vi "Python과 TCP 연결하여 드론 날리기.vi"() -> ()   [LabVIEW 2025]
panel:
  in  "read byte":u32
  in  "port":u32
  in  "localhost":string
  in  "뒤로 플립":bool
  in  "오른쪽 플립":bool
  in  "왼쪽 플립":bool
  in  "우측 회전":bool
  in  "좌측 회전":bool
  in  "하강":bool
  in  "상승":bool
  in  "리턴 홈":bool
  in  "후진":bool
  in  "우측 이동":bool
  in  "좌측 이동":bool
  in  "착륙":bool
  in  "앞으로 플립":bool
  in  "전진":bool
  out "결과":string
  in  "이륙":bool
  in  "종료":bool
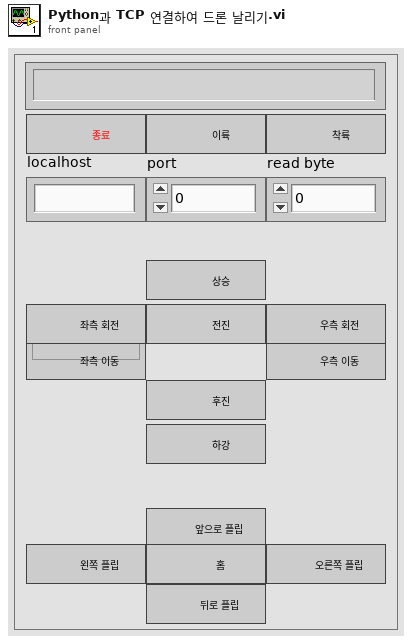
[diagram p1: front panel]
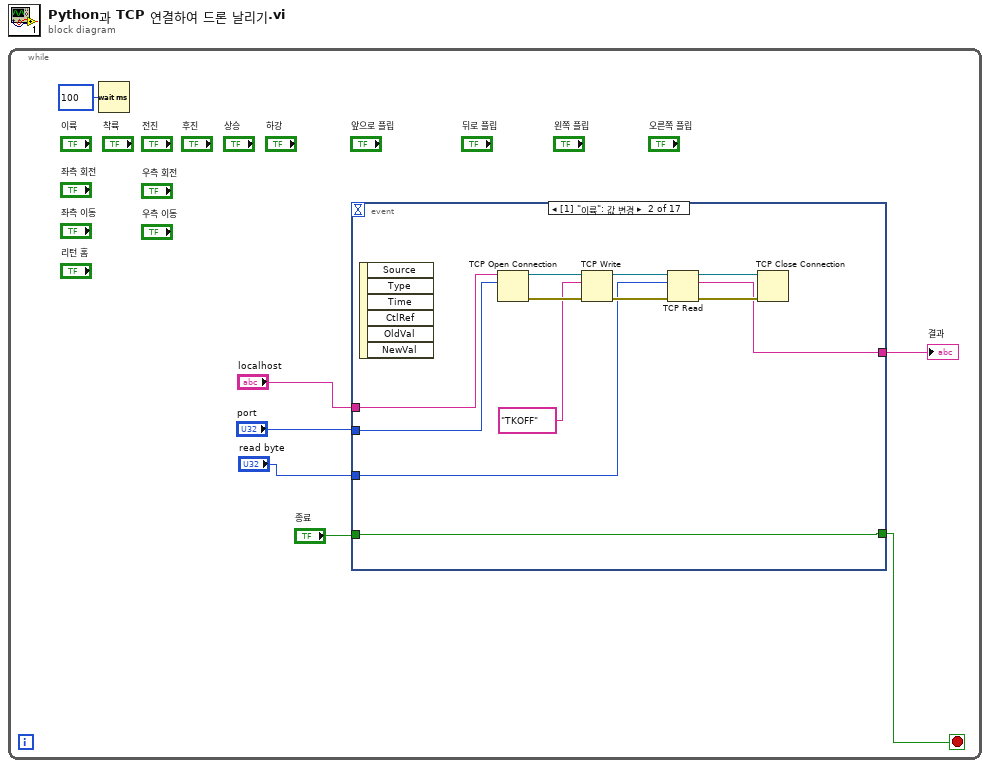
[diagram p0: block diagram]
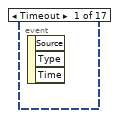
[diagram p2: hidden frame]
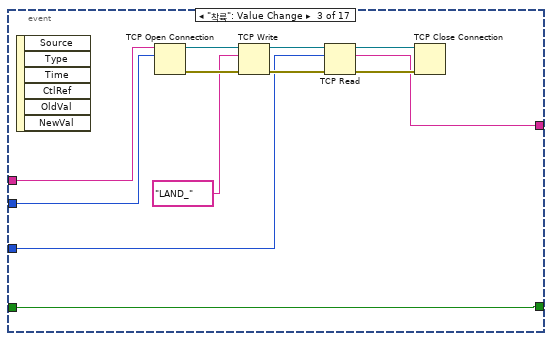
[diagram p3: hidden frame]
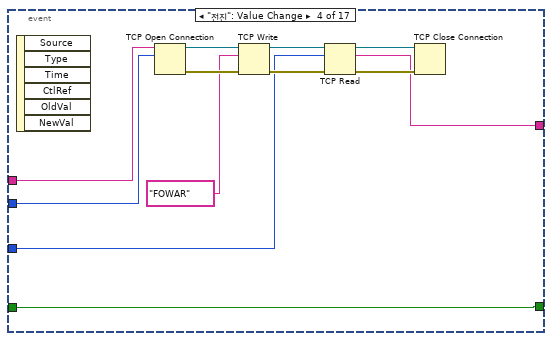
[diagram p4: hidden frame]
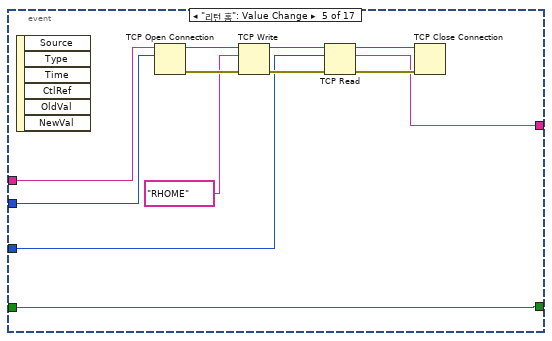
[diagram p5: hidden frame]
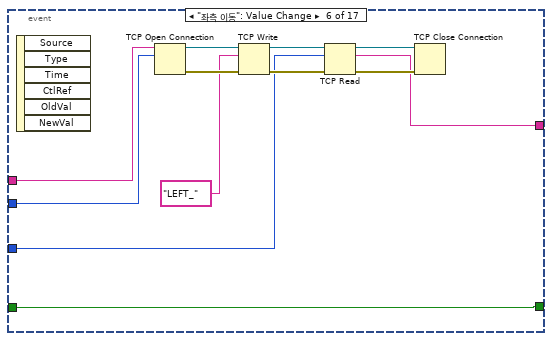
[diagram p6: hidden frame]
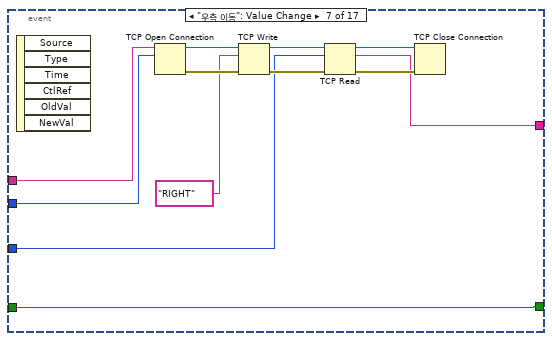
[diagram p7: hidden frame]
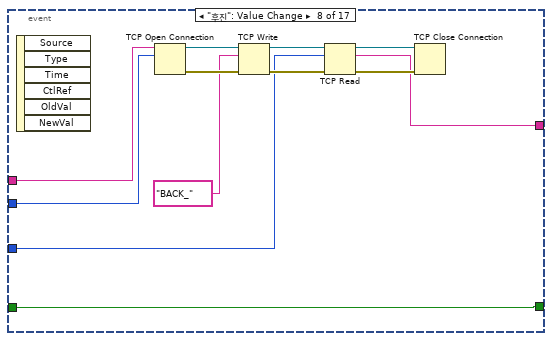
[diagram p8: hidden frame]
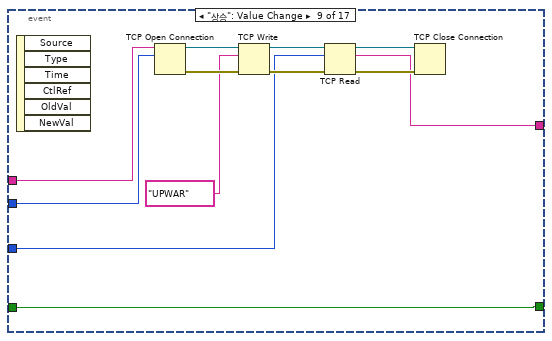
[diagram p9: hidden frame]
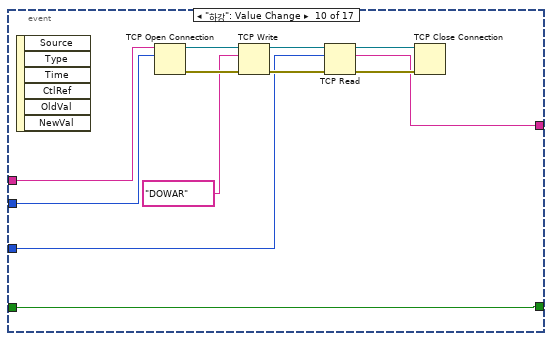
[diagram p10: hidden frame]
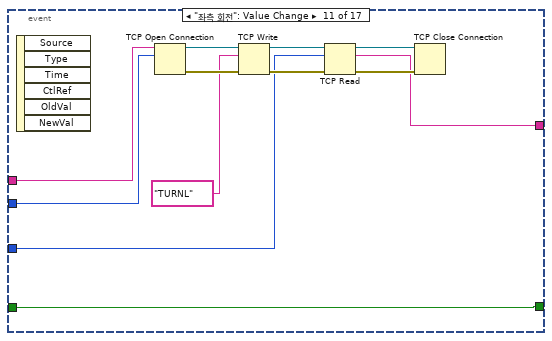
[diagram p11: hidden frame]
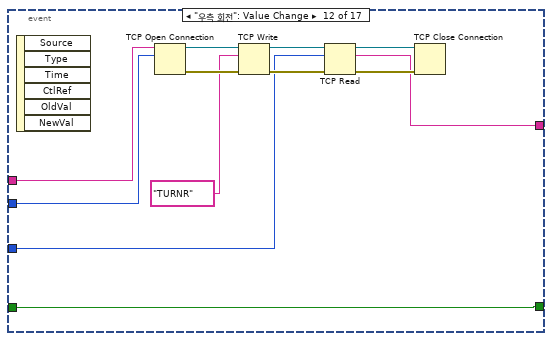
[diagram p12: hidden frame]
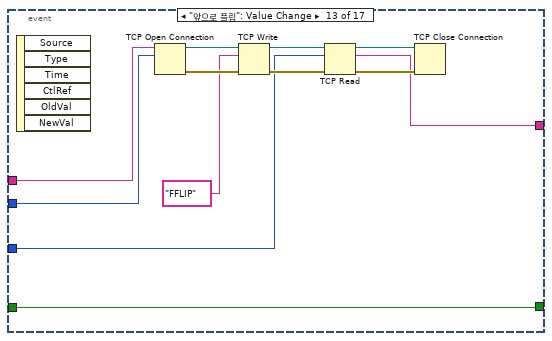
[diagram p13: hidden frame]
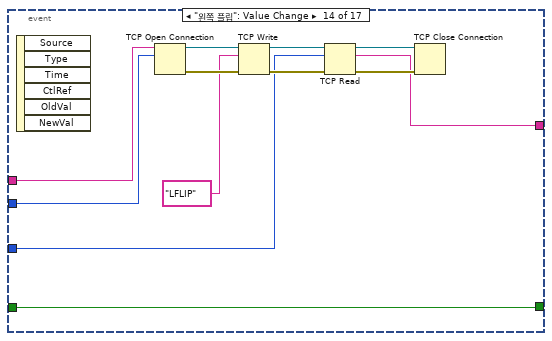
[diagram p14: hidden frame]
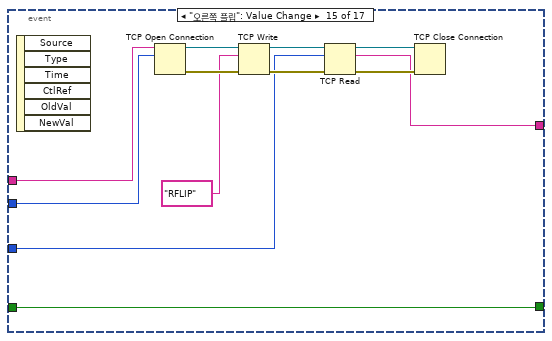
[diagram p15: hidden frame]
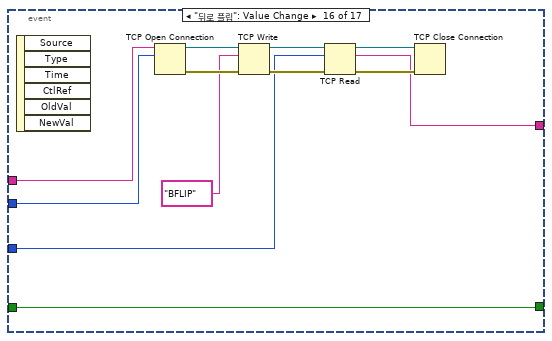
[diagram p16: hidden frame]
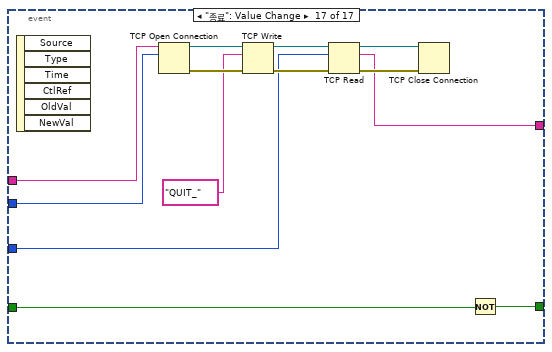
[diagram p17: hidden frame]
diagram:
  n1 = while {
    stop <- w5 stop-if-true
    n2 = Wait (ms)(milliseconds to wait=u32 100 ("대기 시간 (ms)")) -> ()  [unwired: 1 out]
    n3 = event shown="[1] \"이륙\": 값 변경" {
      selector: _ -> [_ _ _ _ _ _ _ _ _ _ _ _ _ _ _ _ _]
      dyn-events: _ -> [_ _ _ _ _ _ _ _ _ _ _ _ _ _ _ _ _]
      timeout: _ -> [_ _ _ _ _ _ _ _ _ _ _ _ _ _ _ _ _]
      tunnel: "localhost" -> [_ w13 w25 w37 w49 w61 w73 w85 w97 w109 w121 w133 w145 w157 w169 w181 w192]
      tunnel: "port" -> [_ w12 w24 w36 w48 w60 w72 w84 w96 w108 w120 w132 w144 w156 w168 w180 w191]
      tunnel: [_ w9 w21 w33 w45 w57 w69 w81 w93 w105 w117 w129 w141 w153 w165 w177 w193] -> w6
      tunnel: "read byte" -> [_ w10 w22 w34 w46 w58 w70 w82 w94 w106 w118 w130 w142 w154 w166 w178 w190]
      tunnel: "종료" -> [_ w8 w20 w32 w44 w56 w68 w80 w92 w104 w116 w128 w140 w152 w164 w176 w189]
      tunnel: [_ w8 w20 w32 w44 w56 w68 w80 w92 w104 w116 w128 w140 w152 w164 w176 w188] -> w5
      event Timeout {
        n4 = event-data() -> ()  [unwired: 1 in, 3 out]
      }
      event "이륙": Value Change {
        n5 = event-data() -> ()  [unwired: 1 in, 6 out]
        n6 = TCP Open Connection(address=w13, remote port or service name=w12) -> (connection ID=w19:refnum<k5>, error out=w16:errorcluster)  [unwired: 3 in]
        n7 = TCP Write(connection ID=w19, data in="TKOFF" ("데이터 입력"), error in (no error)=w16) -> (connection ID out=w18:refnum<k5>, error out=w15:errorcluster)  [unwired: 1 in, 1 out]
        n8 = TCP Read(connection ID=w18, bytes to read=w10, error in (no error)=w15) -> (connection ID out=w17:refnum<k5>, data out=w9:string, error out=w14:errorcluster)  [unwired: 2 in]
        n9 = TCP Close Connection(connection ID=w17, error in (no error)=w14) -> ()  [unwired: 1 in, 2 out]
      }
      event "착륙": Value Change {
        n10 = event-data() -> ()  [unwired: 1 in, 6 out]
        n11 = TCP Open Connection(address=w25, remote port or service name=w24) -> (connection ID=w31:refnum<k5>, error out=w28:errorcluster)  [unwired: 3 in]
        n12 = TCP Write(connection ID=w31, data in="LAND_" ("데이터 입력"), error in (no error)=w28) -> (connection ID out=w30:refnum<k5>, error out=w27:errorcluster)  [unwired: 1 in, 1 out]
        n13 = TCP Read(connection ID=w30, bytes to read=w22, error in (no error)=w27) -> (connection ID out=w29:refnum<k5>, data out=w21:string, error out=w26:errorcluster)  [unwired: 2 in]
        n14 = TCP Close Connection(connection ID=w29, error in (no error)=w26) -> ()  [unwired: 1 in, 2 out]
      }
      event "전진": Value Change {
        n15 = event-data() -> ()  [unwired: 1 in, 6 out]
        n16 = TCP Open Connection(address=w37, remote port or service name=w36) -> (connection ID=w43:refnum<k5>, error out=w40:errorcluster)  [unwired: 3 in]
        n17 = TCP Write(connection ID=w43, data in="FOWAR" ("데이터 입력"), error in (no error)=w40) -> (connection ID out=w42:refnum<k5>, error out=w39:errorcluster)  [unwired: 1 in, 1 out]
        n18 = TCP Read(connection ID=w42, bytes to read=w34, error in (no error)=w39) -> (connection ID out=w41:refnum<k5>, data out=w33:string, error out=w38:errorcluster)  [unwired: 2 in]
        n19 = TCP Close Connection(connection ID=w41, error in (no error)=w38) -> ()  [unwired: 1 in, 2 out]
      }
      event "리턴 홈": Value Change {
        n20 = event-data() -> ()  [unwired: 1 in, 6 out]
        n21 = TCP Open Connection(address=w49, remote port or service name=w48) -> (connection ID=w55:refnum<k5>, error out=w52:errorcluster)  [unwired: 3 in]
        n22 = TCP Write(connection ID=w55, data in="RHOME" ("데이터 입력"), error in (no error)=w52) -> (connection ID out=w54:refnum<k5>, error out=w51:errorcluster)  [unwired: 1 in, 1 out]
        n23 = TCP Read(connection ID=w54, bytes to read=w46, error in (no error)=w51) -> (connection ID out=w53:refnum<k5>, data out=w45:string, error out=w50:errorcluster)  [unwired: 2 in]
        n24 = TCP Close Connection(connection ID=w53, error in (no error)=w50) -> ()  [unwired: 1 in, 2 out]
      }
      event "좌측 이동": Value Change {
        n25 = event-data() -> ()  [unwired: 1 in, 6 out]
        n26 = TCP Open Connection(address=w61, remote port or service name=w60) -> (connection ID=w67:refnum<k5>, error out=w64:errorcluster)  [unwired: 3 in]
        n27 = TCP Write(connection ID=w67, data in="LEFT_" ("데이터 입력"), error in (no error)=w64) -> (connection ID out=w66:refnum<k5>, error out=w63:errorcluster)  [unwired: 1 in, 1 out]
        n28 = TCP Read(connection ID=w66, bytes to read=w58, error in (no error)=w63) -> (connection ID out=w65:refnum<k5>, data out=w57:string, error out=w62:errorcluster)  [unwired: 2 in]
        n29 = TCP Close Connection(connection ID=w65, error in (no error)=w62) -> ()  [unwired: 1 in, 2 out]
      }
      event "우측 이동": Value Change {
        n30 = event-data() -> ()  [unwired: 1 in, 6 out]
        n31 = TCP Open Connection(address=w73, remote port or service name=w72) -> (connection ID=w79:refnum<k5>, error out=w76:errorcluster)  [unwired: 3 in]
        n32 = TCP Write(connection ID=w79, data in="RIGHT" ("데이터 입력"), error in (no error)=w76) -> (connection ID out=w78:refnum<k5>, error out=w75:errorcluster)  [unwired: 1 in, 1 out]
        n33 = TCP Read(connection ID=w78, bytes to read=w70, error in (no error)=w75) -> (connection ID out=w77:refnum<k5>, data out=w69:string, error out=w74:errorcluster)  [unwired: 2 in]
        n34 = TCP Close Connection(connection ID=w77, error in (no error)=w74) -> ()  [unwired: 1 in, 2 out]
      }
      event "후진": Value Change {
        n35 = event-data() -> ()  [unwired: 1 in, 6 out]
        n36 = TCP Open Connection(address=w85, remote port or service name=w84) -> (connection ID=w91:refnum<k5>, error out=w88:errorcluster)  [unwired: 3 in]
        n37 = TCP Write(connection ID=w91, data in="BACK_" ("데이터 입력"), error in (no error)=w88) -> (connection ID out=w90:refnum<k5>, error out=w87:errorcluster)  [unwired: 1 in, 1 out]
        n38 = TCP Read(connection ID=w90, bytes to read=w82, error in (no error)=w87) -> (connection ID out=w89:refnum<k5>, data out=w81:string, error out=w86:errorcluster)  [unwired: 2 in]
        n39 = TCP Close Connection(connection ID=w89, error in (no error)=w86) -> ()  [unwired: 1 in, 2 out]
      }
      event "상승": Value Change {
        n40 = event-data() -> ()  [unwired: 1 in, 6 out]
        n41 = TCP Open Connection(address=w97, remote port or service name=w96) -> (connection ID=w103:refnum<k5>, error out=w100:errorcluster)  [unwired: 3 in]
        n42 = TCP Write(connection ID=w103, data in="UPWAR" ("데이터 입력"), error in (no error)=w100) -> (connection ID out=w102:refnum<k5>, error out=w99:errorcluster)  [unwired: 1 in, 1 out]
        n43 = TCP Read(connection ID=w102, bytes to read=w94, error in (no error)=w99) -> (connection ID out=w101:refnum<k5>, data out=w93:string, error out=w98:errorcluster)  [unwired: 2 in]
        n44 = TCP Close Connection(connection ID=w101, error in (no error)=w98) -> ()  [unwired: 1 in, 2 out]
      }
      event "하강": Value Change {
        n45 = event-data() -> ()  [unwired: 1 in, 6 out]
        n46 = TCP Open Connection(address=w109, remote port or service name=w108) -> (connection ID=w115:refnum<k5>, error out=w112:errorcluster)  [unwired: 3 in]
        n47 = TCP Write(connection ID=w115, data in="DOWAR" ("데이터 입력"), error in (no error)=w112) -> (connection ID out=w114:refnum<k5>, error out=w111:errorcluster)  [unwired: 1 in, 1 out]
        n48 = TCP Read(connection ID=w114, bytes to read=w106, error in (no error)=w111) -> (connection ID out=w113:refnum<k5>, data out=w105:string, error out=w110:errorcluster)  [unwired: 2 in]
        n49 = TCP Close Connection(connection ID=w113, error in (no error)=w110) -> ()  [unwired: 1 in, 2 out]
      }
      event "좌측 회전": Value Change {
        n50 = event-data() -> ()  [unwired: 1 in, 6 out]
        n51 = TCP Open Connection(address=w121, remote port or service name=w120) -> (connection ID=w127:refnum<k5>, error out=w124:errorcluster)  [unwired: 3 in]
        n52 = TCP Write(connection ID=w127, data in="TURNL" ("데이터 입력"), error in (no error)=w124) -> (connection ID out=w126:refnum<k5>, error out=w123:errorcluster)  [unwired: 1 in, 1 out]
        n53 = TCP Read(connection ID=w126, bytes to read=w118, error in (no error)=w123) -> (connection ID out=w125:refnum<k5>, data out=w117:string, error out=w122:errorcluster)  [unwired: 2 in]
        n54 = TCP Close Connection(connection ID=w125, error in (no error)=w122) -> ()  [unwired: 1 in, 2 out]
      }
      event "우측 회전": Value Change {
        n55 = event-data() -> ()  [unwired: 1 in, 6 out]
        n56 = TCP Open Connection(address=w133, remote port or service name=w132) -> (connection ID=w139:refnum<k5>, error out=w136:errorcluster)  [unwired: 3 in]
        n57 = TCP Write(connection ID=w139, data in="TURNR" ("데이터 입력"), error in (no error)=w136) -> (connection ID out=w138:refnum<k5>, error out=w135:errorcluster)  [unwired: 1 in, 1 out]
        n58 = TCP Read(connection ID=w138, bytes to read=w130, error in (no error)=w135) -> (connection ID out=w137:refnum<k5>, data out=w129:string, error out=w134:errorcluster)  [unwired: 2 in]
        n59 = TCP Close Connection(connection ID=w137, error in (no error)=w134) -> ()  [unwired: 1 in, 2 out]
      }
      event "앞으로 플립": Value Change {
        n60 = event-data() -> ()  [unwired: 1 in, 6 out]
        n61 = TCP Open Connection(address=w145, remote port or service name=w144) -> (connection ID=w151:refnum<k5>, error out=w148:errorcluster)  [unwired: 3 in]
        n62 = TCP Write(connection ID=w151, data in="FFLIP" ("데이터 입력"), error in (no error)=w148) -> (connection ID out=w150:refnum<k5>, error out=w147:errorcluster)  [unwired: 1 in, 1 out]
        n63 = TCP Read(connection ID=w150, bytes to read=w142, error in (no error)=w147) -> (connection ID out=w149:refnum<k5>, data out=w141:string, error out=w146:errorcluster)  [unwired: 2 in]
        n64 = TCP Close Connection(connection ID=w149, error in (no error)=w146) -> ()  [unwired: 1 in, 2 out]
      }
      event "왼쪽 플립": Value Change {
        n65 = event-data() -> ()  [unwired: 1 in, 6 out]
        n66 = TCP Open Connection(address=w157, remote port or service name=w156) -> (connection ID=w163:refnum<k5>, error out=w160:errorcluster)  [unwired: 3 in]
        n67 = TCP Write(connection ID=w163, data in="LFLIP" ("데이터 입력"), error in (no error)=w160) -> (connection ID out=w162:refnum<k5>, error out=w159:errorcluster)  [unwired: 1 in, 1 out]
        n68 = TCP Read(connection ID=w162, bytes to read=w154, error in (no error)=w159) -> (connection ID out=w161:refnum<k5>, data out=w153:string, error out=w158:errorcluster)  [unwired: 2 in]
        n69 = TCP Close Connection(connection ID=w161, error in (no error)=w158) -> ()  [unwired: 1 in, 2 out]
      }
      event "오른쪽 플립": Value Change {
        n70 = event-data() -> ()  [unwired: 1 in, 6 out]
        n71 = TCP Open Connection(address=w169, remote port or service name=w168) -> (connection ID=w175:refnum<k5>, error out=w172:errorcluster)  [unwired: 3 in]
        n72 = TCP Write(connection ID=w175, data in="RFLIP" ("데이터 입력"), error in (no error)=w172) -> (connection ID out=w174:refnum<k5>, error out=w171:errorcluster)  [unwired: 1 in, 1 out]
        n73 = TCP Read(connection ID=w174, bytes to read=w166, error in (no error)=w171) -> (connection ID out=w173:refnum<k5>, data out=w165:string, error out=w170:errorcluster)  [unwired: 2 in]
        n74 = TCP Close Connection(connection ID=w173, error in (no error)=w170) -> ()  [unwired: 1 in, 2 out]
      }
      event "뒤로 플립": Value Change {
        n75 = event-data() -> ()  [unwired: 1 in, 6 out]
        n76 = TCP Open Connection(address=w181, remote port or service name=w180) -> (connection ID=w187:refnum<k5>, error out=w184:errorcluster)  [unwired: 3 in]
        n77 = TCP Write(connection ID=w187, data in="BFLIP" ("데이터 입력"), error in (no error)=w184) -> (connection ID out=w186:refnum<k5>, error out=w183:errorcluster)  [unwired: 1 in, 1 out]
        n78 = TCP Read(connection ID=w186, bytes to read=w178, error in (no error)=w183) -> (connection ID out=w185:refnum<k5>, data out=w177:string, error out=w182:errorcluster)  [unwired: 2 in]
        n79 = TCP Close Connection(connection ID=w185, error in (no error)=w182) -> ()  [unwired: 1 in, 2 out]
      }
      event "종료": Value Change {
        n80 = event-data() -> ()  [unwired: 1 in, 6 out]
        n81 = TCP Open Connection(address=w192, remote port or service name=w191) -> (connection ID=w200:refnum<k5>, error out=w197:errorcluster)  [unwired: 3 in]
        n82 = TCP Write(connection ID=w200, data in="QUIT_" ("데이터 입력"), error in (no error)=w197) -> (connection ID out=w199:refnum<k5>, error out=w196:errorcluster)  [unwired: 1 in, 1 out]
        n83 = TCP Read(connection ID=w199, bytes to read=w190, error in (no error)=w196) -> (connection ID out=w198:refnum<k5>, data out=w193:string, error out=w195:errorcluster)  [unwired: 2 in]
        n84 = TCP Close Connection(connection ID=w198, error in (no error)=w195) -> ()  [unwired: 1 in, 2 out]
        n85 = Not(x=w189) -> (.not. x?=w188:bool)
      }
    }
    "결과" <- w6
  }
